vi "Adjust Points.vi"(8 "Previous Point":cluster{"x":dbl, "y":dbl, "th":dbl}, 9 "First Path?":bool, 11 "Points in":cluster{"x":dbl, "y":dbl, "th":dbl}[](array[cluster])) -> (0 "Points out":cluster{"x":dbl, "y":dbl, "th":dbl}[](array[cluster]), 1 "Theta Continuity?":bool, 3 "Next Point":cluster{"x":dbl, "y":dbl, "th":dbl})   [LabVIEW 2025]
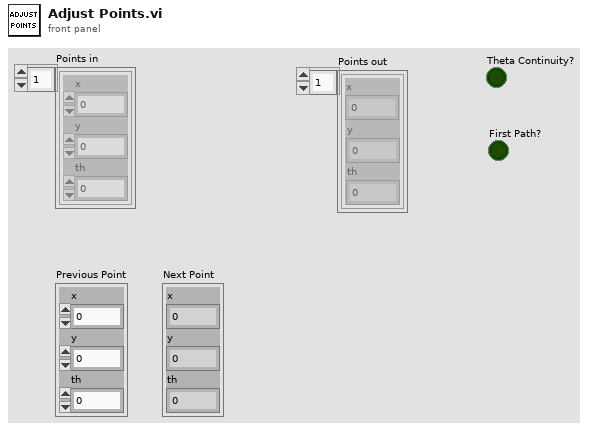
[diagram p1: front panel]
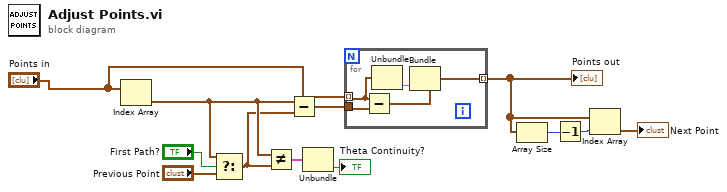
[diagram p0: block diagram]
diagram:
  n1 = Index Array(array="Points in") -> (element=w6:cluster{"x":dbl, "y":dbl, "th":dbl})  [unwired: 1 in]
  n2 = Select(t=w6, s="First Path?", f="Previous Point") -> (s? t:f=w5:cluster{"x":dbl, "y":dbl, "th":dbl})
  n3 = Not Equal?(x=w6, y=w5) -> (x != y?=w10:cluster{"x":bool, "y":bool, "th":bool})
  n4 = Subtract(x=w6, y=w5) -> (x-y=w11:cluster{"x":dbl, "y":dbl, "th":dbl})
  n5 = Unbundle(w10) -> ("th"=→"Theta Continuity?":bool)  [unwired: 2 out]
  n6 = for {
    tunnel: "Points in" -> [w16] mode=indexing
    tunnel: w11 -> [w17]
    tunnel: [w13] -> w3 mode=indexing
    n7 = Subtract(x=w16, y=w17) -> (x-y=w15:cluster{"x":dbl, "y":dbl, "th":dbl})
    n8 = Unbundle(w16) -> ("th"=w14:dbl)  [unwired: 2 out]
    n9 = Bundle(cluster=w15, "th"=w14) -> (w13:cluster{"x":dbl, "y":dbl, "th":dbl})  [unwired: 2 in]
  }
  "Points out" <- w3
  n10 = Array Size(array=w3) -> (size(s)=w4:i32)
  n11 = Decrement(x=w4) -> (x-1=w2:i32)
  n12 = Index Array(array=w3, index=w2) -> (element=→"Next Point":cluster{"x":dbl, "y":dbl, "th":dbl})
